vi "Teleop.vi"(10 "Match Info":T1={"Autonomous Elapsed Seconds"=0.0, "TeleOp Elapsed Seconds"=0.0, "Disabled Elapsed Seconds"=0.0, "Visited Autonomous"=FALSE, "Visited TeleOp"=FALSE, "Visited Disabled"=FALSE, "Autonomous Settings"={"Autonomous Style"=enum."Independent", "VI Refnum"=refnum}}, 11 "Call Context":T2) -> ()   [LabVIEW 2015]
doc: "This VI is called for each TeleOp packet received from the DS where the robot is not disabled. It is often used to read from the joysticks and update I/O or to update setpoints for timed control loops. It should complete and return within 20 milliseconds or it may miss DS packets."
uses:
  <vilib>/Rock Robotics/WPI/DriverStation/WPI_DriverStationDerivedRobotMode.ctl
  <vilib>/Rock Robotics/WPI/DriverStation/WPI_DriverStationMatch Info.ctl
  <vilib>/Rock Robotics/WPI/Utilities/WPI_GetSetVariantRefNum.vi
  <vilib>/Rock Robotics/Network Tables/NT Write Boolean.vi
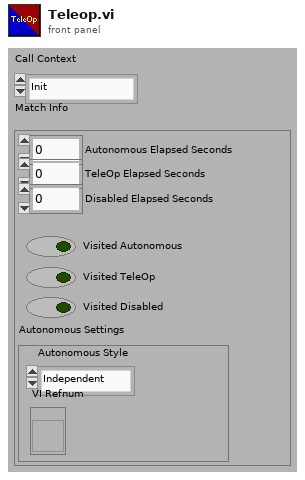
[diagram p1: front panel]
types:
  T1 = typedef "WPI_DriverStationMatch Info.ctl" = cluster{"Autonomous Elapsed Seconds":dbl, "TeleOp Elapsed Seconds":dbl, "Disabled Elapsed Seconds":dbl, "Visited Autonomous":bool, "Visited TeleOp":bool, "Visited Disabled":bool, "Autonomous Settings":cluster{"Autonomous Style":enum16{"Iterative", "Independent"}, "VI Refnum":refnum<vi>}}
  T2 = typedef "WPI_DriverStationDerivedRobotMode.ctl" = enum16{"Init", "Execute", "Stop"}
  T3 = typedef "WPI_JoystickDevRef.ctl" = cluster{"Device":T4}
  T4 = typedef "WPI_JoystickDeviceEnum.ctl" = enum16{"USB 0", "USB 1", "USB 2", "USB 3", "USB 4", "USB 5"}
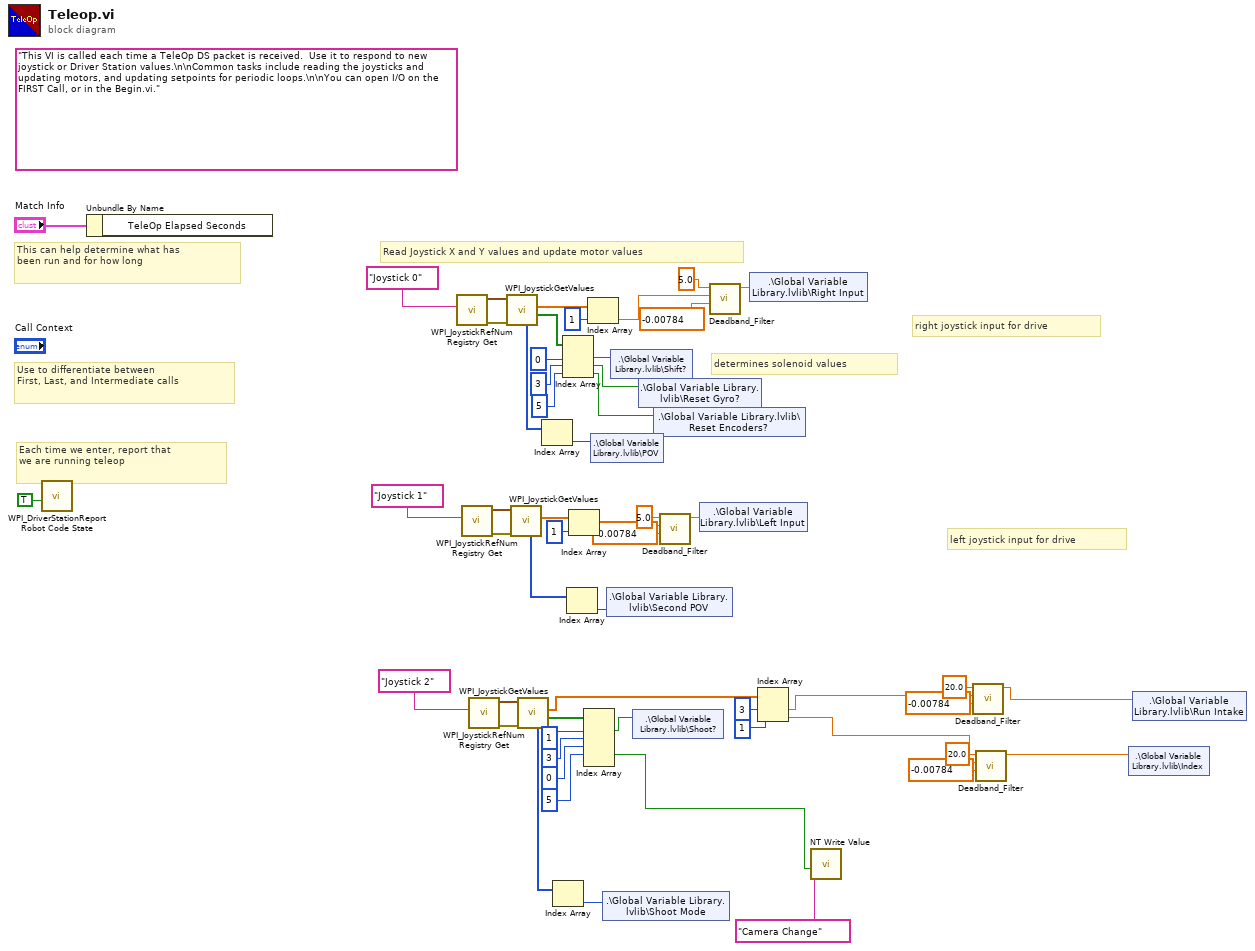
[diagram p0: block diagram]
diagram:
  (unwired) "This VI is called each time a TeleOp DS packet is received.  Use it to respond to new joystick or Driver Station values.\n\nCommon tasks include reading the joysticks and updating motors, and updating setpoints for periodic loops.\n\nYou can open I/O on the FIRST Call, or in the Begin.vi."
  # "left joystick input for drive"
  # "right joystick input for drive"
  # "determines solenoid values"
  # "Each time we enter, report that\nwe are running teleop"
  # "Use to differentiate between\nFirst, Last, and Intermediate calls"
  # "This can help determine what has\nbeen run and for how long"
  # "Read Joystick X and Y values and update motor values"
  n1 = call <vilib>:"WPI_DriverStationReport Robot Code State.vi"("TeleOp"=TRUE ("Autonomous")) -> ()  [unwired: 10 in, 1 out]
  n2 = Unbundle By Name("Match Info") -> ()  [unwired: 1 out]
  n3 = call <vilib>:"WPI_JoystickRefNum Registry Get.vi"("refnum name"="Joystick 0") -> ("error out"=w50:errorcluster, "JoystickDevRef"=w49:T3)  [unwired: 1 in, 8 out]
  n4 = call <vilib>:"WPI_JoystickRefNum Registry Get.vi"("refnum name"="Joystick 1") -> ("error out"=w43:errorcluster, "JoystickDevRef"=w42:T3)  [unwired: 1 in, 8 out]
  n5 = call <vilib>:"WPI_JoystickRefNum Registry Get.vi"("refnum name"="Joystick 2") -> ("error out"=w40:errorcluster, "JoystickDevRef"=w39:T3)  [unwired: 1 in, 8 out]
  n6 = call <vilib>:"WPI_JoystickGetValues.vi"("error in (no error)"=w50, "JoystickDevRef"=w49) -> ("Buttons"=w47:bool[], "Axes"=w48:dbl[], "POVs"=w45:i16[])  [unwired: 5 in, 2 out]
  n7 = call <vilib>:"WPI_JoystickGetValues.vi"("error in (no error)"=w43, "JoystickDevRef"=w42) -> ("Axes"=w41:dbl[], "POVs"=w22:i16[])  [unwired: 5 in, 3 out]
  n8 = call <vilib>:"WPI_JoystickGetValues.vi"("error in (no error)"=w40, "JoystickDevRef"=w39) -> ("Buttons"=w38:bool[], "Axes"=w18:dbl[], "POVs"=w25:i16[])  [unwired: 5 in, 2 out]
  n9 = Index Array(array=w45) -> (element=w44:i16)  [unwired: 1 in]
  n10 = Index Array(array=w25) -> (element=w24:i16)  [unwired: 1 in]
  n11 = Index Array(array=w47, index #1=0 ("index"), index #2=3 ("index"), index #3=5 ("index")) -> (element #1=w46:bool, element #2=w23:bool, element #3=w3:bool)
  n12 = Index Array(array=w22) -> (element=w21:i16)  [unwired: 1 in]
  n13 = Index Array(array=w41, index=1) -> (element=w31:dbl)
  n14 = Index Array(array=w38, index #1=1 ("index"), index #2=3 ("index"), index #3=0 ("index"), index #4=5 ("index")) -> (element #1=w37:bool, element #4=w6:bool)  [unwired: 1 in, 3 out]
  n15 = Index Array(array=w48, index=1) -> (element=w26:dbl)
  n16 = shared-variable ".\\Global Variable Library.lvlib\\POV"(w44) -> ()  [unwired: 1 in, 1 out]
  n17 = shared-variable ".\\Global Variable Library.lvlib\\Shoot Mode"(w24) -> ()  [unwired: 1 in, 1 out]
  n18 = shared-variable ".\\Global Variable Library.lvlib\\Second POV"(w21) -> ()  [unwired: 1 in, 1 out]
  n19 = shared-variable ".\\Global Variable Library.lvlib\\Shift?"(w46) -> ()  [unwired: 1 in, 1 out]
  n20 = shared-variable ".\\Global Variable Library.lvlib\\Shoot?"(w37) -> ()  [unwired: 1 in, 1 out]
  n21 = shared-variable ".\\Global Variable Library.lvlib\\Reset Gyro?"(w23) -> ()  [unwired: 1 in, 1 out]
  n22 = shared-variable ".\\Global Variable Library.lvlib\\Reset Encoders?"(w3) -> ()  [unwired: 1 in, 1 out]
  n23 = call "Deadband_Filter.vi"("Deadband_Center"=-0.00784, "Input"=w31, "Deadband_Size(%)"=5.0) -> ("Deadbanded_Output"=w1:dbl)  [unwired: 8 in]
  n24 = shared-variable ".\\Global Variable Library.lvlib\\Left Input"(w1) -> ()  [unwired: 1 in, 1 out]
  n25 = call "Deadband_Filter.vi"("Deadband_Center"=-0.00784, "Input"=w26, "Deadband_Size(%)"=5.0) -> ("Deadbanded_Output"=w2:dbl)  [unwired: 8 in]
  n26 = shared-variable ".\\Global Variable Library.lvlib\\Right Input"(w2) -> ()  [unwired: 1 in, 1 out]
  n27 = Index Array(array=w18, index #1=3 ("index"), index #2=1 ("index")) -> (element #1=w11:dbl, element #2=w8:dbl)
  n28 = call-poly <vilib>:"NT Write Value.vi"("Boolean"=w6, "Name"="Camera Change") -> ()  [unwired: 9 in, 1 out]
  n29 = call "Deadband_Filter.vi"("Deadband_Center"=-0.00784, "Input"=w11, "Deadband_Size(%)"=20.0) -> ("Deadbanded_Output"=w12:dbl)  [unwired: 8 in]
  n30 = call "Deadband_Filter.vi"("Deadband_Center"=-0.00784, "Input"=w8, "Deadband_Size(%)"=20.0) -> ("Deadbanded_Output"=w7:dbl)  [unwired: 8 in]
  n31 = shared-variable ".\\Global Variable Library.lvlib\\Index"(w7) -> ()  [unwired: 1 in, 1 out]
  n32 = shared-variable ".\\Global Variable Library.lvlib\\Run Intake"(w12) -> ()  [unwired: 1 in, 1 out]
